vi "convert_pressure_CCP.vi"(7 "conv_type":enum16{"None", "Torr2psig"}(ring), 11 "P_in":dbl) -> (3 "P_out":dbl)   [LabVIEW 2019]
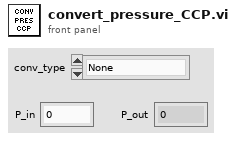
[diagram p1: front panel]
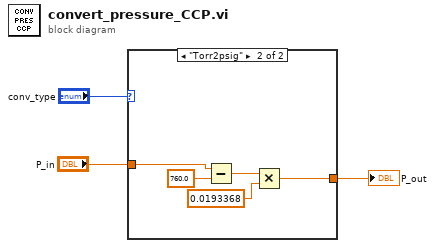
[diagram p0: block diagram]
diagram:
  n1 = case shown="\"Torr2psig\"" "conv_type" {
    tunnel: "P_in" -> [w4 w8]
    tunnel: [w4 w5] -> w1
    frame "None", Default {
    }
    frame "Torr2psig" {
      n2 = Subtract(x=w8, y=760.0) -> (x-y=w7:dbl)
      n3 = Multiply(x=w7, y=0.0193368) -> (x*y=w5:dbl)
    }
  }
  "P_out" <- w1
